vi "Binary MLS (obs 90).vi"(2 "seed":i64=-1 format="%.0x", 3 "polynomial order":i32=31 max=512, 4 "samples":i64=128) -> (0 "error code":i32, 1 "mls sequence":u8[](array[numeric]))   [LabVIEW 2010, in "NI_AALBase.lvlib"]
doc: "The Binary MLS VI was rewritten in LabVIEW 2009. Replace this VI with a Binary MLS VI from the <B>Functions</B> palette to use the new functionality.\n\nGenerates a maximum length sequence of ones and zeroes using a modulo-2 primitive polynomial of order <B>polynomial order</B>."
uses:
  NI_AALBase.lvlib
panel:
  # "Binary MLS"
  # "This VI is obsolete !!!\nYou should replace this VI in your diagram with the Binary MLS VI."
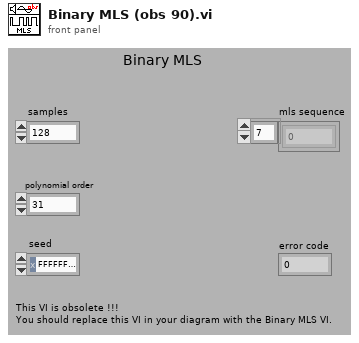
[diagram p1: front panel]
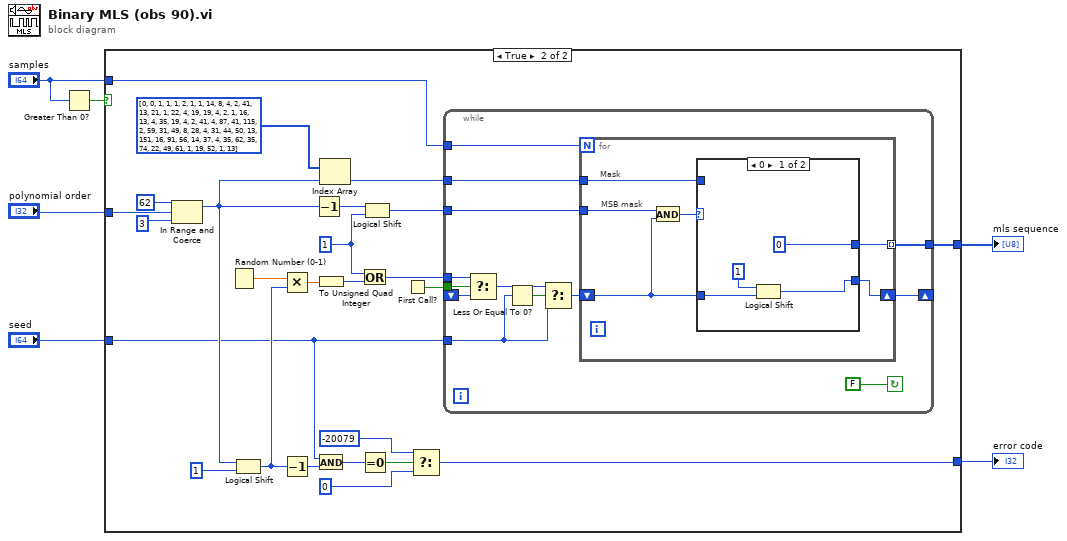
[diagram p0: block diagram]
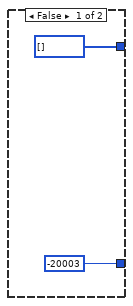
[diagram p2: hidden frame]
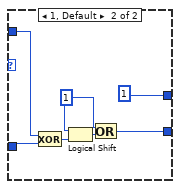
[diagram p3: hidden frame]
diagram:
  n1 = Greater Than 0?(x="samples") -> (x > 0?=w1:bool)
  n2 = case shown="True" w1 {
    tunnel: "polynomial order" -> [_ w31]
    tunnel: "samples" -> [_ w27]
    tunnel: [u8[] [] w24] -> w5
    tunnel: [-20003 ("t") w18] -> w4
    tunnel: "seed" -> [_ w10]
    frame False {
    }
    frame True {
      w9 = u64 1 ("y")
      n3 = In Range and Coerce(upper limit=u16 62, x=w31, lower limit=u16 3) -> (coerced(x)=w21:i32)  [unwired: 1 out]
      n4 = Random Number (0-1)() -> (number: 0 to 1=w13:dbl)
      n5 = Logical Shift(y=w21, x=u64 1 ("y")) -> (x << y=w12:u64)
      n6 = Multiply(x=w13, y=w12) -> (x*y=w15:dbl)
      n7 = Decrement(x=w12) -> (x-1=w22:u64)
      n8 = Decrement(x=w21) -> (x-1=w28:i32)
      n9 = To Unsigned Quad Integer(1:w15) -> (0:w14:u64)
      n10 = And(x=w10, y=w22) -> (x .and. y?=w25:u64)
      n11 = Index Array(array=u64[] [0, 0, 1, 1, 1, 2, 1, 1, 14, 8, 4, 2, 41, 13, 21, 1, 22, 4, 19, 19, 4, 2, 1, 16, 13, 4, 35, 19, 4, 2, 41, 4, 87, 41, 115, 2, 59, 31, 49, 8, 28, 4, 31, 44, 50, 13, 151, 16, 91, 56, 14, 37, 4, 35, 62, 35, 74, 22, 49, 61, 1, 19, 52, 1, 13] ("appended array"), index=w21) -> (element=w30:u64)
      n12 = Or(x=w9, y=w14) -> (x .or. y?=w11:u64)
      n13 = Equal To 0?(x=w25) -> (x = 0?=w20:bool)
      n14 = Logical Shift(y=w28, x=w9) -> (x << y=w29:u64)
      n15 = First Call?() -> (First Call?: T/F=w16:bool)
      n16 = Select(t=-20079, s=w20, f=0) -> (s? t:f=w18:i32)
      n17 = while {
        tunnel: w30 -> [w46]
        tunnel: w29 -> [w45]
        tunnel: w11 -> [w37]
        tunnel: w27 -> [w44]
        tunnel: [w43] -> w24
        tunnel: w10 -> [w34]
        tunnel: w16 -> [w38]
        shift-right: [w39] -> _
        shift-left: _ -> [w36]
        stop <- FALSE continue-if-true
        n18 = Select(t=w37, s=w38, f=w36) -> (s? t:f=w35:u64)
        n19 = Less Or Equal To 0?(x=w34) -> (x <= 0?=w40:bool)
        n20 = Select(t=w35, s=w40, f=w34) -> (s? t:f=w41:u64)
        n21 = for {
          N: w44 -> [_]
          shift-right: [w50] -> w39
          shift-left: w41 -> [w47]
          tunnel: w46 -> [w52]
          tunnel: w45 -> [w51]
          tunnel: [w48] -> w43 mode=indexing
          # "MSB mask"
          # "Mask"
          n22 = And(x=w51, y=w47) -> (x .and. y?=w49:u64)
          n23 = case shown="0" w49 {
            tunnel: w47 -> [w56 w62]
            tunnel: w52 -> [_ w63]
            tunnel: [w54 w59] -> w50
            tunnel: [u8 0 ("y") u8 1 ("y")] -> w48
            frame 0 {
              n24 = Logical Shift(y=u32 1, x=w56) -> (x << y=w54:u64)
            }
            frame 1, Default {
              w58 = u64 1 ("y")
              n25 = Exclusive Or(1:w62, 2:w63) -> (0:w61:u64)
              n26 = Logical Shift(y=w58, x=w61) -> (x << y=w60:u64)
              n27 = Or(x=w58, y=w60) -> (x .or. y?=w59:u64)
            }
          }
        }
      }
    }
  }
  "mls sequence" <- w5
  "error code" <- w4
